vi "TCC.vi"(0 "Porta Medidor":refnum<visa-resource-name>) -> ()   [LabVIEW 2009]
doc: "The Advanced Serial Read and Write example performs a Serial Port Read, a Serial Port Write, or a combination of these actions while setting some advanced serial features like buffer size, termination characters, and XON/XOFF flow control. The user selects the actions (read or write) on the front panel. If both are selected, the VI will write the data first, read the data and then close the VISA session that is opened to the port. \n\nThe parameters set for the serial port must match the parameters of the connected instrument or device. In this example, the bytes to read parameter specifies the number of bytes that the serial port reads. If there were more bytes at the port than the number specified in bytes to read, those bytes would not be read. Also, if you specify to read more bytes than the number of bytes actually read, you might receive a timeout error message.\n\nINSTRUCTIONS:\n1) Select the serial resource and configuration parameters (baud rate, data bits, parity, stop bits, flow control).\n2) Termination character can be enabled and set. Also, set the required input buffer size prior to running the example.\n3) Select the operations to be performed. \n4) Connect the serial port to your device. If no device is available, perform a loopback test by doing one of the following. Short pins 2 and 3 on a RS-232 cable or short pin 4 to pin 8 and pin 5 to pin 9 on a RS-485/422 cable. \n5) Run the VI to see the data read. (The \"read string\" will match the \"string to write\" if a loopback test was performed.)\n\nThis example exposes several advanced features that you may need for your application. Not all applications need all the features shown in this example. The input buffer size is likely an important setting that you want to control in your application. This example expands upon the flow control option for XON and XOFF, allowing the user to choose those control characters. The timeout parameter has been brought to the front panel so a user can specify the time period the VISA Read will wait for the number of bytes to read before timing out. Also, the user has several controls for the termination character, which is discussed later.\n\nNote that you can press the write and read buttons and change the bytes to read parameters on the fly, while the example is running. However, you must stop the example to change the other configuration parameters after the example has started running, and then run again.\n\nSet the I/O buffer size slightly higher the amount of data you expect to receive. This is very important for applications that don't use flow control, as you may lose characters if the receive buffer overflows.\n\nSetting the timeout period ensures that the operation returns with a timeout error if the operation cannot be performed in the specified time period. \n\nSome devices require a termination character in order to identify the end of command strings. Some devices send a termination character to signify the end of data to be read. \n\nThis example shows how you can end the Read operation once a termination character is detected in the buffer and/or append a termination character at the end of the Write data. To enable the Read to end on a termination character, use the VISA Configure Serial Port or use the VISA Properties Serial End Mode for Reads, Termination Character Enable, and Termination Character. To end the Write with a termination character, use the VISA Properties Serial End Mode for Writes, the Send End Enable, and Termination Character. In this example, the same termination character is used for both the Read and the Write. You can specify two different characters for your application, if desired.\n\nYour application may require specific characters for the XON/XOFF Flow Control. You can specify these characters with the VISA Properties Flow Control XOFF Character and Flow Control XON Character. Note that if the standard XON and XOFF characters are used, then decimal 17 and 19 are unavailable for data values. Remember that using flow control and setting an adequate buffer size allow you to prevent buffer overflows."
uses:
  <vilib>/Instr/_visa.llb/VISA Configure Serial Port (Instr).vi
panel:
  out "Erro Médio (%)":dbl
  out "Erro Máximo (%)":dbl
  out "Erro (%)":dbl
  out "Rotação\nTacômetro (RPM)":dbl format="%#_6f"
  in  "Porta Tacômetro":refnum<visa-resource-name>
  out "Forma de Onda":cluster{dbl, dbl}(graph)
  out "Rotação\nMedidor (RPM)":dbl format="%#_6f"
  in  "stop":bool
  # "Medidor de rotação a partir da análise da corrente de excitação\nComparativo"
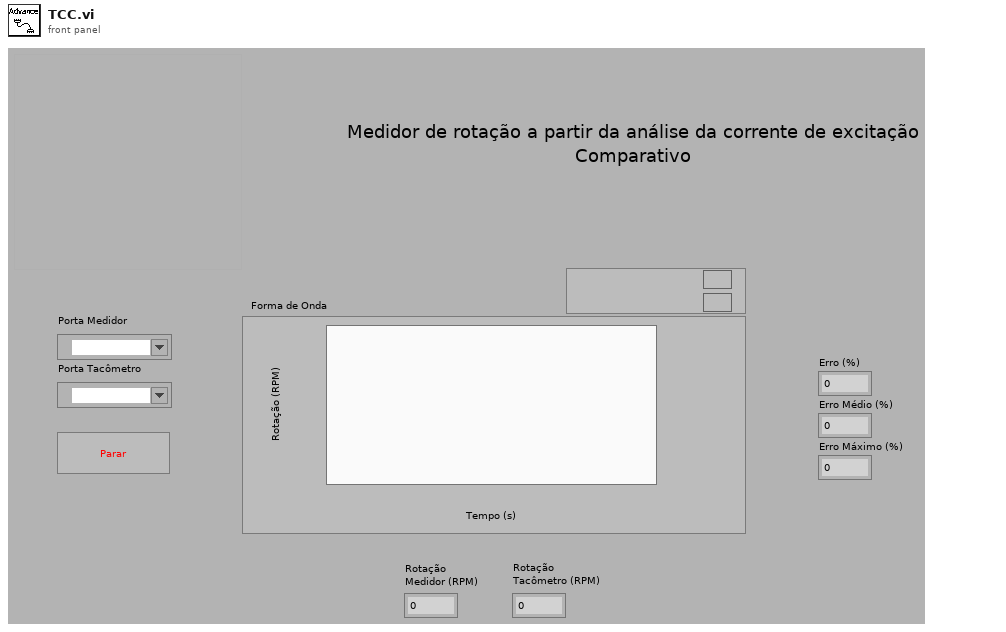
[diagram p1: front panel]
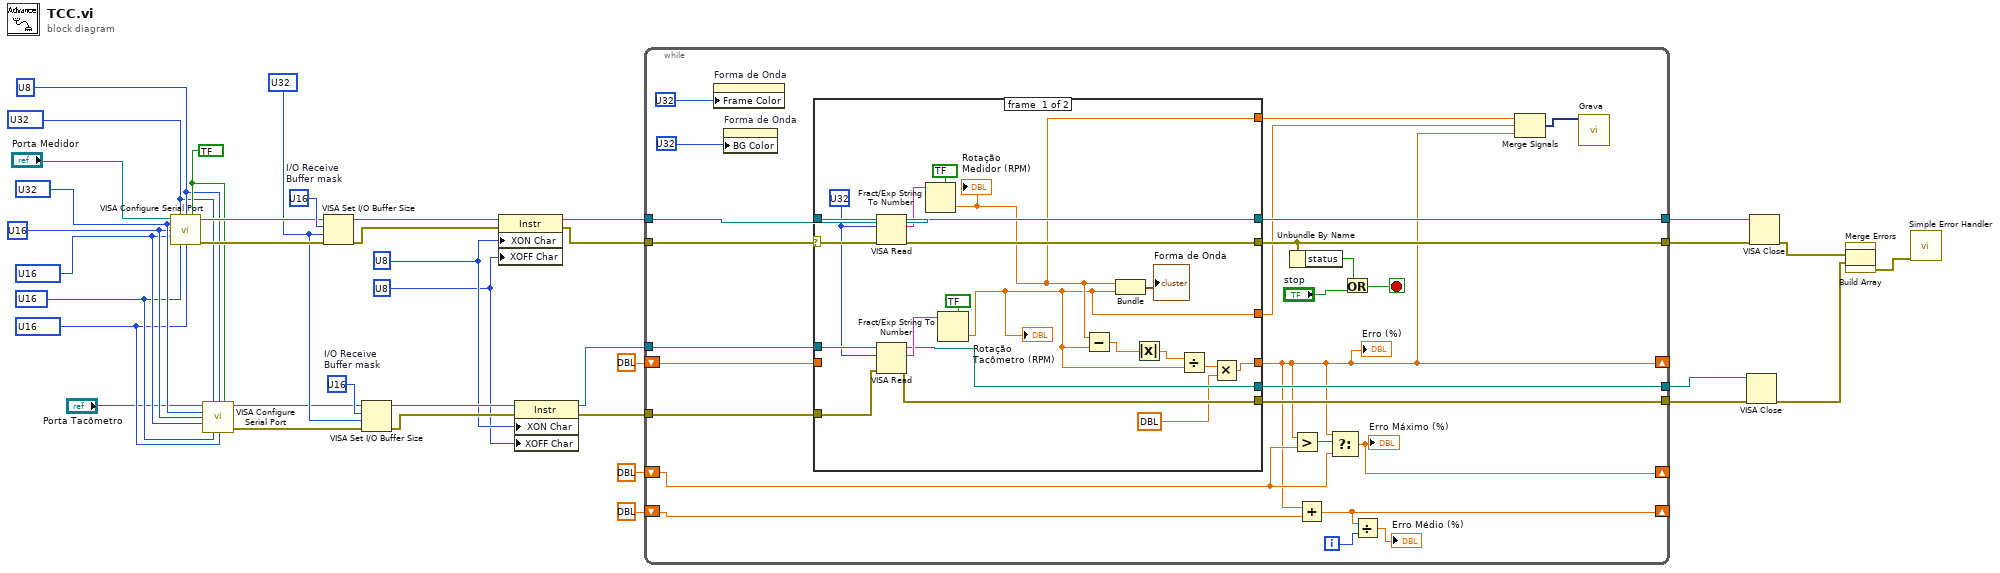
[diagram p0: block diagram]
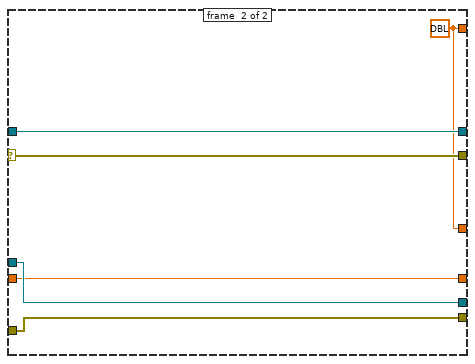
[diagram p2: hidden frame]
diagram:
  w16 = u32 ? ("Input\nbuffer size")
  w28 = bool ? ("End read on termination character?")
  w12 = u8 ? ("XOFF Character")
  w13 = u8 ? ("XON Character")
  w21 = u16 ? items=["None", "XON/XOFF", "RTS/CTS", "DTR/DSR"] ("flow control")
  w22 = u16 ? items=["1.0", "1.5", "2.0"] ("stop bits")
  w23 = u16 ? items=["None", "Odd", "Even", "Mark", "Space"] ("parity")
  w26 = u32 ? ("timeout (ms)")
  w27 = u8 ? ("termination char\n(0xA = '\\n' = LF)")
  w24 = u16 ? ("data bits")
  w25 = u32 ? ("baud rate")
  w17 = u16 ?  # I/O Receive Buffer mask
  w37 = u16 ?  # I/O Receive Buffer mask
  n1 = call-poly "VISA Configure Serial Port"("VISA resource name"="Porta Medidor", "timeout (10sec)"=w26, "termination char\n(0xA = '\\n' = LF)"=w27, "Enable Termination\nChar (T)"=w28, "baud rate (9600)"=w25, "data bits (8)"=w24, "parity (0:none)"=w23, "stop bits (10: 1 bit)"=w22, "flow control (0:none)"=w21) -> ("VISA resource name out"=w30:refnum<visa-resource-name>, "error out"=w29:errorcluster)  [unwired: 5 in]
  n2 = call-poly "VISA Configure Serial Port"("VISA resource name"="Porta Tacômetro", "timeout (10sec)"=w26, "termination char\n(0xA = '\\n' = LF)"=w27, "Enable Termination\nChar (T)"=w28, "baud rate (9600)"=w25, "data bits (8)"=w24, "parity (0:none)"=w23, "stop bits (10: 1 bit)"=w22, "flow control (0:none)"=w21) -> ("VISA resource name out"=w15:refnum<visa-resource-name>, "error out"=w14:errorcluster)  [unwired: 5 in]
  n3 = VISA Set I/O Buffer Size(VISA resource name=w30, mask (16)=w37, size (4096)=w16, error in (no error)=w29) -> (VISA resource name out=w36:refnum<visa-resource-name>, error out=w35:errorcluster)
  n4 = VISA Set I/O Buffer Size(VISA resource name=w15, mask (16)=w17, size (4096)=w16, error in (no error)=w14) -> (VISA resource name out=w18:refnum<visa-resource-name>, error out=w19:errorcluster)
  n5 = property class="Instr"(reference=w36, error in=w35, "XON Char"=w13, "XOFF Char"=w12) -> (reference out=w33:refnum<visa-resource-name>, error out=w34:errorcluster)
  n6 = property class="Instr"(reference=w18, error in=w19, "XON Char"=w13, "XOFF Char"=w12) -> (reference out=w11:refnum<visa-resource-name>, error out=w10:errorcluster)
  n7 = while {
    tunnel: w34 -> [w57]
    tunnel: w33 -> [w58]
    tunnel: [w62] -> w32
    tunnel: [w61] -> w31
    tunnel: w11 -> [w56]
    tunnel: w10 -> [w55]
    tunnel: [w54] -> w6
    tunnel: [w53] -> w5
    shift-right: [w40] -> _
    shift-left: dbl ? -> [w49]
    shift-right: [w45] -> _
    shift-left: dbl ? -> [w48]
    shift-right: [w44] -> _
    shift-left: dbl ? -> [w43]
    i -> [w46]
    stop <- w60 stop-if-true
    n8 = property on="Forma de Onda" class="WFChart (strict)"("Frame Color"=u32 ?) -> ()  [unwired: 2 in, 2 out]
    n9 = property on="Forma de Onda" class="WFChart (strict)"("BG Color"=u32 ?) -> ()  [unwired: 2 in, 2 out]
    n10 = case "Read bytes from port." shown="Error" w57 {
      selector: w57 -> [w82 w89]
      tunnel: [w74 w89] -> w61
      tunnel: [w84 w90] -> w62
      tunnel: w58 -> [w83 w90]
      tunnel: w56 -> [w78 w88]
      tunnel: w55 -> [w77 w87]
      tunnel: [w73 w88] -> w54
      tunnel: [w72 w87] -> w53
      tunnel: [w66 w86] -> w40
      tunnel: w49 -> [_ w86]
      tunnel: [w65 w85] -> w42
      tunnel: [w64 w85] -> w41
      frame #0 {
        w76 = u32 ? ("bytes to read")
        n11 = VISA Read(VISA resource name=w83, byte count=w76, error in (no error)=w82) -> (VISA resource name out=w84:refnum<visa-resource-name>, read buffer=w81:string, error out=w74:errorcluster)  [unwired: 1 out]
        n12 = VISA Read(VISA resource name=w78, byte count=w76, error in (no error)=w77) -> (VISA resource name out=w73:refnum<visa-resource-name>, read buffer=w75:string, error out=w72:errorcluster)  [unwired: 1 out]
        n13 = Fract/Exp String To Number(use system decimal point (T)=bool ?, string=w81) -> (number=w65:dbl)  [unwired: 2 in, 1 out]
        "Rotação\nMedidor (RPM)" <- w65
        n14 = Fract/Exp String To Number(use system decimal point (T)=bool ?, string=w75) -> (number=w64:dbl)  [unwired: 2 in, 1 out]
        "Rotação\nTacômetro (RPM)" <- w64
        n15 = Subtract(x=w65, y=w64) -> (x-y=w69:dbl)
        n16 = Bundle(w65, w64) -> (→"Forma de Onda":cluster{dbl, dbl})  [unwired: 1 in]
        n17 = Absolute Value(x=w69) -> (abs(x)=w70:dbl)
        n18 = Divide(x=w70, y=w64) -> (x/y=w68:dbl)
        n19 = Multiply(x=w68, y=dbl ?) -> (x*y=w66:dbl)
      }
      frame #1 {
        w85 = dbl ?
      }
    }
    "Erro (%)" <- w40
    n20 = Unbundle By Name(w61) -> ("status"=w63:bool)
    n21 = Greater?(x=w40, y=w43) -> (0:w50:bool)
    n22 = Add(x=w40, y=w48) -> (x+y=w45:dbl)
    n23 = Select(t=w40, s=w50, f=w43) -> (s? t:f=w44:dbl)
    "Erro Máximo (%)" <- w44
    n24 = Or(x=w63, y="stop") -> (x .or. y?=w60:bool)
    n25 = Divide(x=w45, y=w46) -> (x/y=→"Erro Médio (%)":dbl)
    n26 = Merge Signals(w42, w41, w40) -> (w39:dynamicdata)
    n27 = call "Grava"("Signals"=w39) -> ()  [unwired: 16 in, 3 out]
  }
  n28 = VISA Close(VISA resource name=w6, error in (no error)=w5) -> (error out=w8:errorcluster)
  n29 = VISA Close(VISA resource name=w32, error in (no error)=w31) -> (error out=w9:errorcluster)
  n30 = Build Array(w9, w8) -> (w1:errorcluster[])
  n31 = call <vilib>:"Merge Errors.vi"("error array in"=w1) -> ("error out"=w7:errorcluster)  [unwired: 6 in]
  n32 = call <vilib>:"Simple Error Handler.vi"("error in (no error)"=w7) -> ()  [unwired: 4 in, 5 out]
